vi "myRIO v1.0 Configure I2C.vi"(8 "error in (no error)":errorcluster, 9 "I2C Counter Value":u8, 10 "Channel":T1, 11 "myRIO Ref In":T2) -> (0 "error out":errorcluster, 3 "myRIO Ref Out":T2)   [LabVIEW 2021]
uses:
  <vilib>/myRIO/Common/Instrument Driver Framework/Utilities/typedefs/myRIO v1.0 Reference.ctl
  <vilib>/myRIO/Common/Instrument Driver Framework/Utilities/typedefs/Generic FPGA Reference.ctl
  <vilib>/myRIO/Common/Instrument Driver Framework/myRIO v1.0/I2C/typedefs/I2C Channels Enum.ctl
  <vilib>/myRIO/Common/Instrument Driver Framework/myRIO v1.0/I2C/typedefs/I2C Channels FPGA Reference.ctl
  <vilib>/rvi/errors/niLvFpgaAdjustHostInterfaceError.vi
  <vilib>/rvi/interface/nirviReadWriteControl/nirviReadWriteControl.xnode
  <vilib>/rvi/interface/Simulation/niFpgaSimulationCallBeginRW.vi
  NiFpgaLv.dll
panel:
  # "This VI configures the I2C counter register (I2C.n_0.CNTR) based on the value of the I2C Transfer Rate control and sets bit 0 of the configuration register (I2C.n_0.CNFG) to enable the I2C master logic in the FPGA.\nPlease see Block Diagram for details."
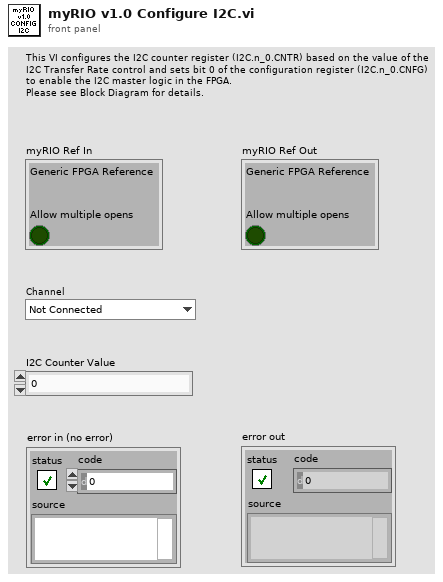
[diagram p1: front panel]
types:
  T1 = typedef "I2C Channels Enum.ctl" = enum16{"Not Connected", "A/I2C", "B/I2C", "I2C/I2C"}
  T2 = typedef "myRIO v1.0 Reference.ctl" = cluster{"Generic FPGA Reference":T3, "Allow multiple opens":bool}
  T3 = typedef "Generic FPGA Reference.ctl" = refnum<k20>
  T4 = typedef "I2C Channels FPGA Reference.ctl" = refnum<k20>
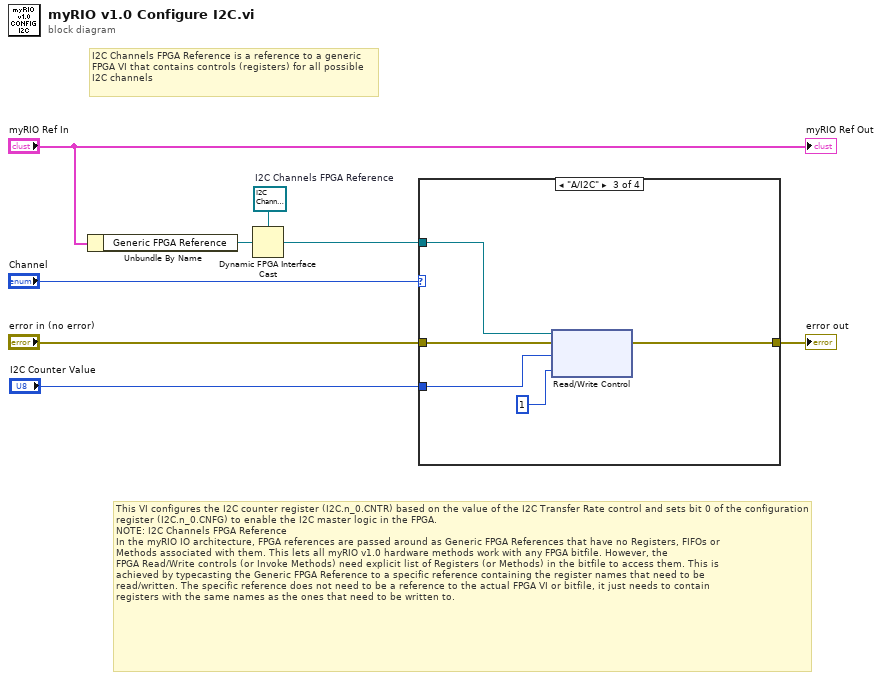
[diagram p0: block diagram]
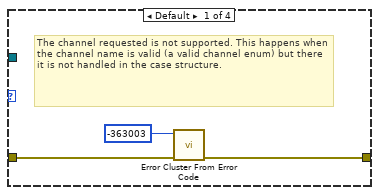
[diagram p2: hidden frame]
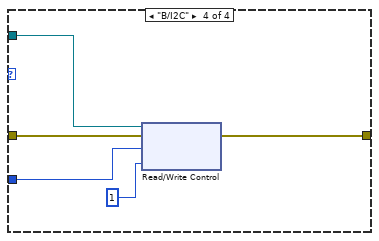
[diagram p4: hidden frame]
diagram:
  w8 = T4 refnum  # I2C Channels FPGA Reference
  # "This VI configures the I2C counter register (I2C.n_0.CNTR) based on the value of the I2C Transfer Rate control and sets bit 0 of the configuration register (I2C.n_0.CNFG) to enable the I2C master logic in the FPGA.\nNOTE: I2C Channels FPGA Reference\nIn the myRIO IO architecture, FPGA references are passed around as Generic FPGA References that have no Registers, FIFOs or\nMethods associated with them. This lets all myRIO v1.0 hardware methods work with any FPGA bitfile. However, the \nFPGA Read/Write controls (or Invoke Methods) need explicit list of Registers (or Methods) in the bitfile to access them. This is \nachieved by typecasting the Generic FPGA Reference to a specific reference containing the register names that need to be \nread/written. The specific reference does not need to be a reference to the actual FPGA VI or bitfile, it just needs to contain \nregisters with the same names as the ones that need to be written to."
  # "I2C Channels FPGA Reference is a reference to a generic FPGA VI that contains controls (registers) for all possible I2C channels"
  n1 = Unbundle By Name("myRIO Ref In") -> ("Generic FPGA Reference"=w1:T3)
  n2 = Dynamic FPGA Interface Cast(Session In=w8, Type=w1) -> (Session Out=w7:T4)
  n3 = case shown="\"A/I2C\"" "Channel" {
    tunnel: "error in (no error)" -> [w9 w12 w16 w21]
    tunnel: [w10 w12 w15 w20] -> w4
    tunnel: w7 -> [_ _ w17 w22]
    tunnel: "I2C Counter Value" -> [_ _ w13 w19]
    frame Default {
      # "The channel requested is not supported. This happens when the channel name is valid (a valid channel enum) but there it is not handled in the case structure."
      n4 = call <vilib>:"Error Cluster From Error Code.vi"("error in (no error)"=w9, "error code (0)"=-363003) -> ("error out"=w10:errorcluster)  [unwired: 7 in]
    }
    frame "Not Connected" {
    }
    frame "A/I2C" {
      n5 = xnode "Read/Write Control"("FPGA VI Reference In"=w17, "error in"=w16, "I2C.A.CNTR"=w13, "I2C.A.CNFG"=u8 1 ("I2C0.CNFG")) -> ("error out"=w15:errorcluster)  [unwired: 1 out]
    }
    frame "B/I2C" {
      n6 = xnode "Read/Write Control"("FPGA VI Reference In"=w22, "error in"=w21, "I2C.B.CNTR"=w19, "I2C.B.CNFG"=u8 1 ("I2C0.CNFG")) -> ("error out"=w20:errorcluster)  [unwired: 1 out]
    }
  }
  "error out" <- w4
  "myRIO Ref Out" <- "myRIO Ref In"
